vi "Protocol.Create Protocol Settings.vi"(8 "error in (no error)":errorcluster, 10 "Name in":string, 11 "Parameters in":T4={"XNET Settings"={"Database"="", "Cluster"="", "Port"="", "Baud rate [Bd]"=0, "Termination"=0, "Incoming Rate"=0, "Outcoming Rate"=1, "Write Decimation"=1}, "Data"=[], "DTCs"=[], "Sim Addresses LUT"=variant, "Data Table LUT"=variant, "MonitorTool.Network"={"Address"=0, "Name"=0}, "Name"=""} {"MonitorTool.Network"."Name" format="%.0x"; "DTCs"."Data"."DM1 Ref"."Data Reference" format="%.0x"; "DTCs"."Data"."DM1 Enable Ref"."Data Reference" format="%.0x"; "DTCs"."Data"."DM2 Ref"."Data Reference" format="%.0x"; "DTCs"."Data"."DM2 Enable Ref"."Data Reference" format="%.0x"; "Data"."Network"."Name" format="%.0x"; "Data"."IncomingRefs"."Data Reference" format="%.0x"; "Data"."OutgoingRefs"."Data Reference" format="%.0x"; "XNET Settings"."Termination" items=["Off", "On"]}) -> (0 "error out":errorcluster, 3 "Protocol Refs":T1)   [LabVIEW 2015, in "J1939 Addon Engine.lvlib"]
uses:
  J1939 Addon Engine.lvlib
  Types/Protocol.App Settings.ctl
  Shared/Types/XNET Settings.ctl
  Types/Protocol.XNET Refs.ctl
  <vilib>/NI Veristand/Custom Device API/Block Data Reference.ctl
  <vilib>/NI Veristand/Custom Device API/Data Reference.ctl
  Shared/Types/Monitor Settings.ctl
  Types/Engine.DTC Settings.ctl
  Shared/Types/Compiled Simulated Settings.ctl
  Types/Engine.DTC FIFOs.ctl
  Types/Protocol.Refs.ctl
  Shared/J1939 Utilities/Types/CAN Outgoing Message Cluster.ctl
  Types/Protocol.RQST Lookup Table Reference.ctl
  Types/Protocol.Address Table Reference.ctl
  Shared/J1939 Utilities/J1939 Utilities.lvlib
  Shared/J1939 Addon Shared.lvlib
  <vilib>/NI VeriStand/Custom Device API/Custom Device API.lvlib
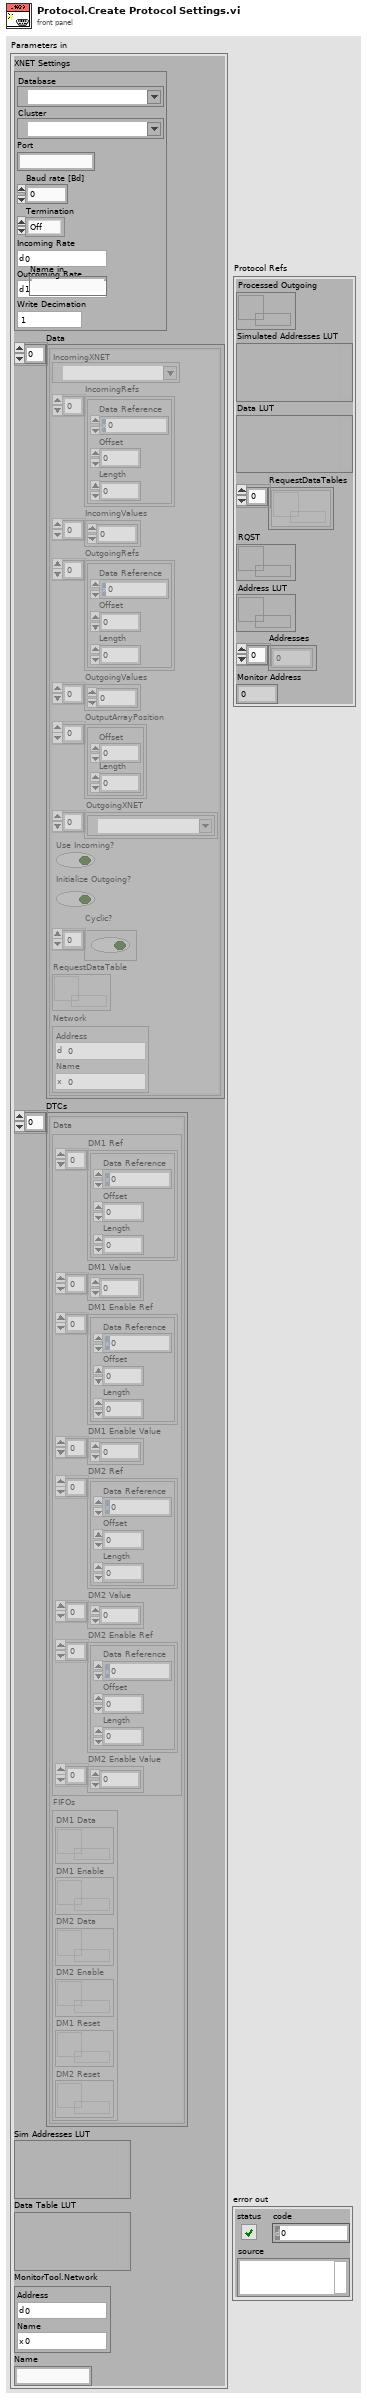
[diagram p1: front panel]
types:
  T1 = typedef "J1939 Addon Engine.lvlib/Protocol.Refs.ctl" = cluster{"Processed Outgoing":refnum<queue>, "Simulated Addresses LUT":variant, "Data LUT":variant, "RequestDataTables":refnum<k33>[], "RQST":T2, "Address LUT":T3, "Addresses":u8[], "Monitor Address":u8}
  T2 = typedef "J1939 Addon Engine.lvlib/Protocol.RQST Lookup Table Reference.ctl" = refnum<data-value>
  T3 = typedef "J1939 Addon Engine.lvlib/Protocol.Address Table Reference.ctl" = refnum<data-value>
  T4 = typedef "J1939 Addon Engine.lvlib/Protocol.App Settings.ctl" = cluster{"XNET Settings":T5, "Data":T6[], "DTCs":T10[], "Sim Addresses LUT":variant, "Data Table LUT":variant, "MonitorTool.Network":T9, "Name":string}
  T5 = typedef "J1939 Addon Shared.lvlib/XNET Settings.ctl" = cluster{"Database":refnum<k21>, "Cluster":refnum<k21>, "Port":string, "Baud rate [Bd]":u32, "Termination":u32, "Incoming Rate":u32, "Outcoming Rate":u32, "Write Decimation":u32}
  T6 = typedef "J1939 Addon Engine.lvlib/Protocol.XNET Refs.ctl" = cluster{"IncomingXNET":refnum<k21>, "IncomingRefs":T7[], "IncomingValues":dbl[], "OutgoingRefs":T7[], "OutgoingValues":dbl[], "OutputArrayPosition":cluster{"Offset":u32, "Length":u32}[], "OutgoingXNET":refnum<k21>[], "Use Incoming?":bool, "Initialize Outgoing?":bool, "Cyclic?":bool[], "RequestDataTable":refnum<k33>, "Network":T9}
  T7 = typedef "Custom Device API.lvlib/Block Data Reference.ctl" = cluster{"Data Reference":T8, "Offset":u64, "Length":u64}
  T8 = typedef "Custom Device API.lvlib/Data Reference.ctl" = i32
  T9 = typedef "J1939 Addon Shared.lvlib/Monitor Settings.ctl" = cluster{"Address":u8, "Name":u64}
  T10 = typedef "J1939 Addon Engine.lvlib/Engine.DTC Settings.ctl" = cluster{"Data":T11, "FIFOs":T12}
  T11 = typedef "J1939 Addon Shared.lvlib/Compiled Simulated Settings.ctl" = cluster{"DM1 Ref":T7[], "DM1 Value":dbl[], "DM1 Enable Ref":T7[], "DM1 Enable Value":dbl[], "DM2 Ref":T7[], "DM2 Value":dbl[], "DM2 Enable Ref":T7[], "DM2 Enable Value":dbl[]}
  T12 = typedef "J1939 Addon Engine.lvlib/Engine.DTC FIFOs.ctl" = cluster{"DM1 Data":refnum<k33>, "DM1 Enable":refnum<k33>, "DM2 Data":refnum<k33>, "DM2 Enable":refnum<k33>, "DM1 Reset":refnum<k33>, "DM2 Reset":refnum<k33>}
  T13 = typedef "J1939 Addon Shared.lvlib/J1939 Utilities.lvlib/CAN Outgoing Message Cluster.ctl" = cluster{"Identifier":u32, "Data":u8[]}
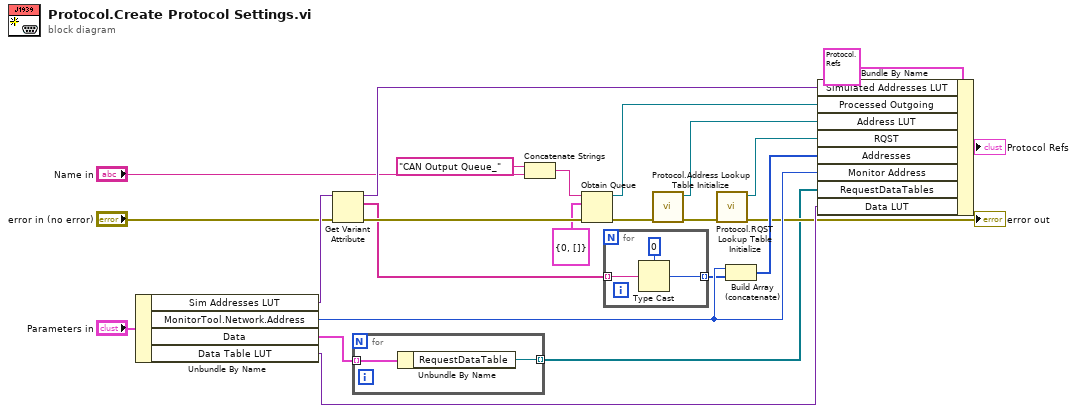
[diagram p0: block diagram]
diagram:
  n1 = Unbundle By Name("Parameters in") -> ("Sim Addresses LUT"=w20:variant, "MonitorTool.Network.Address"=w24:u8, "Data"=w22:T6[], "Data Table LUT"=w21:variant)
  n2 = Get Variant Attribute(Variant=w20, error in="error in (no error)") -> (duplicate Variant=w23:variant, names=w2:string[], error out=w19:errorcluster)  [unwired: 2 in, 1 out]
  n3 = for {
    tunnel: w22 -> [w26] mode=indexing
    tunnel: [w25] -> w1 mode=indexing
    n4 = Unbundle By Name(w26) -> ("RequestDataTable"=w25:refnum<k33>)
  }
  n5 = Concatenate Strings("CAN Output Queue_" ("name (unnamed)"), "Name in") -> (w10:string)
  n6 = Obtain Queue(name (unnamed)=w10, element data type=T13 {"Identifier"=0, "Data"=[]} ("Data to Send"), error in (no error)=w19) -> (queue out=w12:refnum<queue>, error out=w4:errorcluster)  [unwired: 2 in, 1 out]
  n7 = for {
    tunnel: w2 -> [w29] mode=indexing
    tunnel: [w27] -> w3 mode=indexing
    n8 = Type Cast(type=u8 0, x=w29) -> (*(type *) &x=w27:u8)
  }
  n9 = call "Protocol.Address Lookup Table Initialize.vi"("error in (no error)"=w4) -> ("error out"=w5:errorcluster, "Address LUT"=w13:T3)  [unwired: 9 in]
  n10 = call "Protocol.RQST Lookup Table Initialize.vi"("error in (no error)"=w5) -> ("error out"=→"error out":errorcluster, "Rqst LUT"=w14:T2)  [unwired: 9 in]
  n11 = Build Array (concatenate)(w24, w3) -> (w15:u8[])
  n12 = Bundle By Name(cluster=T1 {"Processed Outgoing"=refnum, "Simulated Addresses LUT"=variant, "Data LUT"=variant, "RequestDataTables"=[], "RQST"=refnum, "Address LUT"=refnum, "Addresses"=[], "Monitor Address"=0} ("Protocol Refs"), "Simulated Addresses LUT"=w23, "Processed Outgoing"=w12, "Address LUT"=w13, "RQST"=w14, "Addresses"=w15, "Monitor Address"=w24, "RequestDataTables"=w1, "Data LUT"=w21) -> (→"Protocol Refs":T1)
